vi "Insert Start Message.vi"(8 "error in (no error)":errorcluster, 10 "Start Time":timestamp, 11 "Electrophysiology in":refnum<class "Electrophysiology.lvclass">) -> (0 "error out":errorcluster, 3 "Electrophysiology out":refnum<class "Electrophysiology.lvclass">)   [LabVIEW 2014, in "Electrophysiology.lvclass"]
uses:
  Electrophysiology.lvclass
  Database/EphysPrimary.ctl
  Database/SessionPrimary.ctl
  AcquireTraces/AcquireTraces.lvclass
  AcquistionObject/AcquistionObject.lvclass
panel:
  out "EphysPK":T1
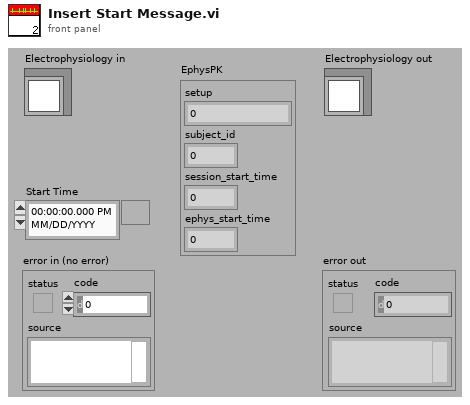
[diagram p1: front panel]
types:
  T1 = typedef "EphysPrimary.ctl" = cluster{"setup":u8, "subject_id":i32, "session_start_time":dbl, "ephys_start_time":dbl}
  T2 = cluster{"setup":u8, "subject_id":i32, "session_start_time":dbl, "ephys_start_time":dbl, "ephys_path":path, "ephys_task":string, "ephys_stop_time":dbl}
  T3 = typedef "NI_Database_API.lvlib/Conn ObjectReference.ctl" = refnum<k1>
  T4 = typedef "SessionPrimary.ctl" = cluster{"setup":u8, "subject_id":i32, "session_start_time":dbl}
  T5 = cluster{"reference":T3, "table":string, "columns":string[], i32}
  T6 = cluster{cluster{"reference":T3, "table":string, "columns":string[], i32}, "Variant":variant}
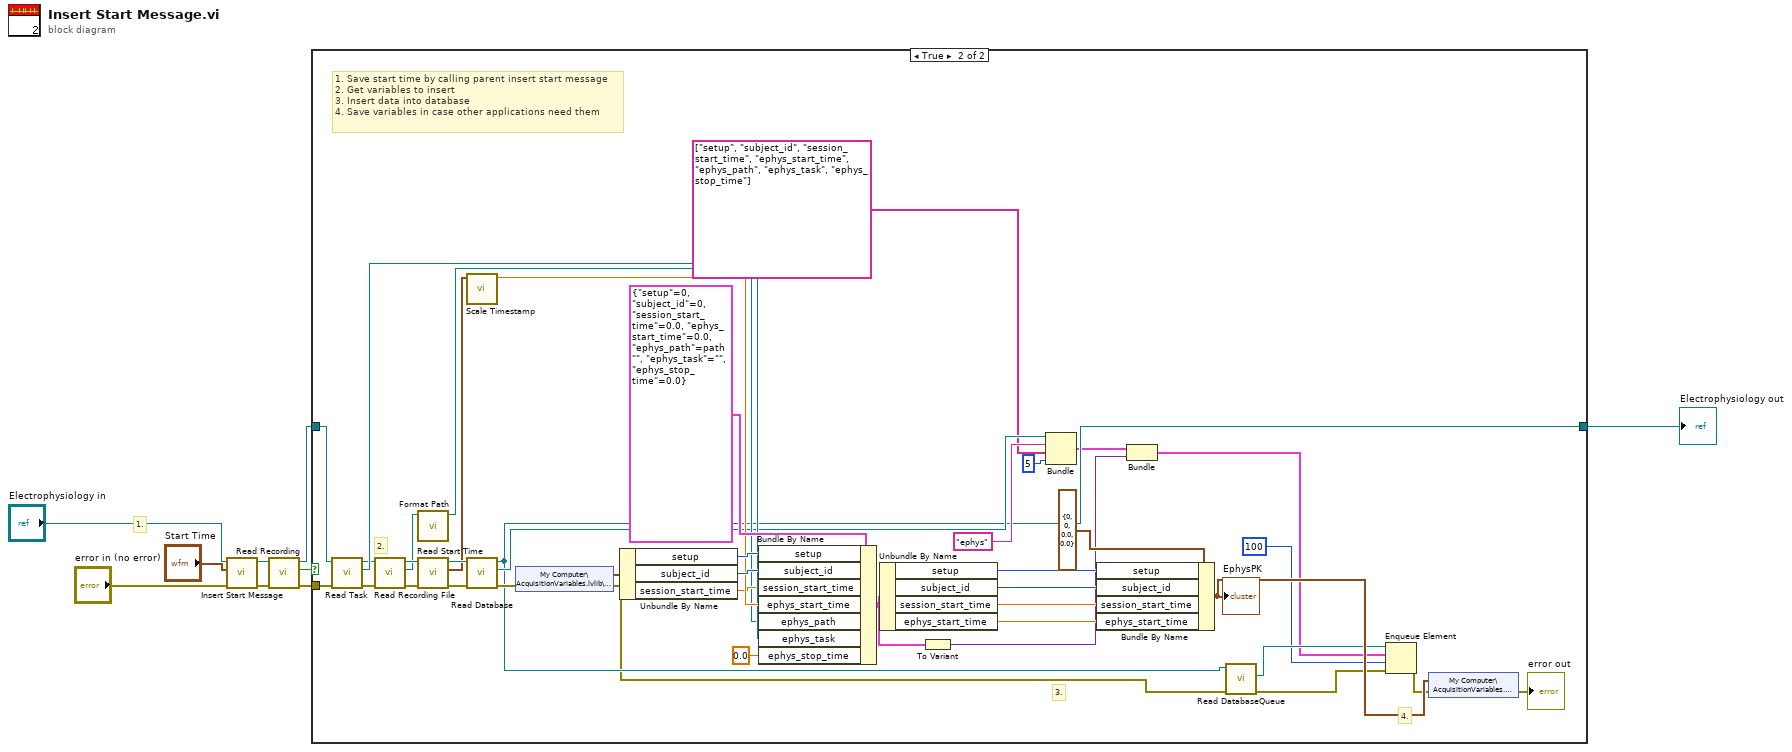
[diagram p0: block diagram]
diagram:
  # "1."
  n1 = call-parent "Insert Start Message.vi"("error in (no error)"="error in (no error)", "Start Time"="Start Time", "AcquireTraces in"="Electrophysiology in") -> ("error out"=w5:errorcluster, "AcquireTraces out"=w6:refnum<class "Electrophysiology.lvclass">)  [unwired: 7 in]
  n2 = call-dynamic "Read Recording.vi"("error in (no error)"=w5, "AcquireTraces in"=w6) -> ("error out"=w3:errorcluster, "Recording"=w4:bool, "AcquireTraces out"=w2:refnum<class "Electrophysiology.lvclass">)  [unwired: 7 in]
  n3 = case shown="True" w4 {
    tunnel: w3 -> [_ w31]
    tunnel: w2 -> [w10 w33]
    tunnel: [w10 w22] -> w1
    frame False {
    }
    frame True {
      # "4."
      # "2."
      # "3."
      # "1. Save start time by calling parent insert start message\n2. Get variables to insert\n3. Insert data into database\n4. Save variables in case other applications need them"
      n4 = call-dynamic "Read Task.vi"("error in (no error)"=w31, "AcquireTraces in"=w33) -> ("error out"=w30:errorcluster, "Task"=w34:refnum<k21>, "AcquireTraces out"=w32:refnum<class "Electrophysiology.lvclass">)  [unwired: 7 in]
      n5 = call-dynamic "Read Recording File.vi"("error in (no error)"=w30, "AcquistionObject in"=w32) -> ("error out"=w41:errorcluster, "Recording File"=w27:path, "AcquistionObject out"=w42:refnum<class "Electrophysiology.lvclass">)  [unwired: 7 in]
      n6 = call "Format Path.vi"("Input path"=w27) -> ("Output path"=w26:path)  [unwired: 10 in]
      n7 = call-dynamic "Read Start Time.vi"("error in (no error)"=w41, "AcquistionObject in"=w42) -> ("error out"=w39:errorcluster, "Start Time"=w36:timestamp, "AcquistionObject out"=w40:refnum<class "Electrophysiology.lvclass">)  [unwired: 7 in]
      n8 = call "Scale Timestamp.vi"("Time Stamp"=w36) -> ("Scaled timestamp"=w35:dbl)  [unwired: 10 in]
      n9 = call-dynamic "Read Database.vi"("error in (no error)"=w39, "AcquistionObject in"=w40) -> ("error out"=w38:errorcluster, "reference"=w25:T3, "AcquistionObject out"=w22:refnum<class "Electrophysiology.lvclass">)  [unwired: 7 in]
      n10 = shared-variable "My Computer\\AcquisitionVariables.lvlib\\SessionPK"(error in=w38) -> (w44:T4, error out=w21:errorcluster)
      n11 = Unbundle By Name(w44) -> ("setup"=w50:u8, "subject_id"=w49:i32, "session_start_time"=w29:dbl)
      n12 = Bundle By Name(cluster=T2 {"setup"=0, "subject_id"=0, "session_start_time"=0.0, "ephys_start_time"=0.0, "ephys_path"=path "", "ephys_task"="", "ephys_stop_time"=0.0} ("Cluster"), "setup"=w50, "subject_id"=w49, "session_start_time"=w29, "ephys_start_time"=w35, "ephys_path"=w26, "ephys_task"=w34, "ephys_stop_time"=0.0) -> (w13:T2)
      n13 = Unbundle By Name(w13) -> ("setup"=w47:u8, "subject_id"=w46:i32, "session_start_time"=w28:dbl, "ephys_start_time"=w45:dbl)
      n14 = To Variant(anything=w13) -> (Variant=w14:variant)
      n15 = Bundle("reference"=w25, "table"="ephys", "columns"=string[] ["setup", "subject_id", "session_start_time", "ephys_start_time", "ephys_path", "ephys_task", "ephys_stop_time"], 5) -> (w15:T5)  [unwired: 1 in]
      n16 = Bundle By Name(cluster=T1 {"setup"=0, "subject_id"=0, "session_start_time"=0.0, "ephys_start_time"=0.0} ("EphysPK"), "setup"=w47, "subject_id"=w46, "session_start_time"=w28, "ephys_start_time"=w45) -> (w43:T1)
      "EphysPK" <- w43
      n17 = Bundle(w15, "Variant"=w14) -> (w12:T6)  [unwired: 1 in]
      n18 = call-dynamic "Read DatabaseQueue.vi"("error in (no error)"=w21, "AcquistionObject in"=w22) -> ("error out"=w20:errorcluster, "DatabaseQueue"=w18:refnum<queue>)  [unwired: 7 in, 1 out]
      n19 = Enqueue Element(queue=w18, element=w12, timeout in ms (-1)=100, error in (no error)=w20) -> (error out=w19:errorcluster)  [unwired: 2 out]
      n20 = shared-variable "My Computer\\AcquisitionVariables.lvlib\\EphysPK"(w43, error in=w19) -> (error out=→"error out":errorcluster)
    }
  }
  "Electrophysiology out" <- w1
